vi "readBoardCounts.vi"(2 "input_portNum":i32=2, 3 "VISA resource name":refnum<visa-resource-name>="COM1") -> (0 "show_countInRange":bool=TRUE, 1 "show_messageOut":string="Port0 Usage Frequency: 017\nPort1 Usage Frequency: 017")   [LabVIEW 2011]
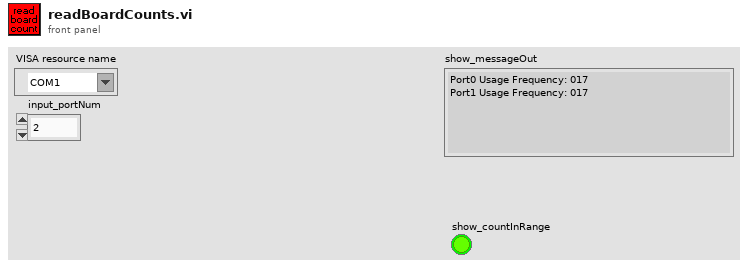
[diagram p1: front panel]
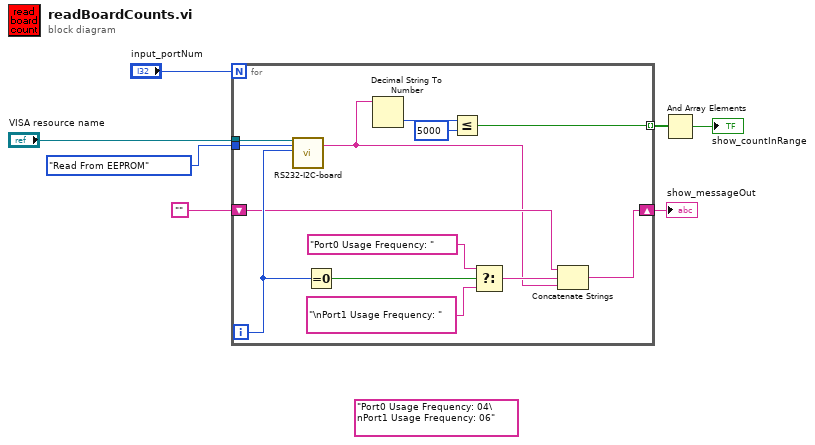
[diagram p0: block diagram]
diagram:
  (unwired) "Port0 Usage Frequency: 04\nPort1 Usage Frequency: 06"
  n1 = for {
    N: "input_portNum" -> [_]
    tunnel: "VISA resource name" -> [w20]
    tunnel: enum16{"Write to EEPROM", "Read From EEPROM"}."Read From EEPROM" ("Function") -> [w19]
    shift-right: [w12] -> w3
    shift-left: "" -> [w13]
    tunnel: [w8] -> w2 mode=indexing
    i -> [w18]
    n2 = call "RS232-I2C-board.vi"("VISA resource name"=w20, "Function"=w19, "Select channel"=w18) -> ("Read Data"=w11:string)  [unwired: 10 in, 6 out]
    n3 = Equal To 0?(x=w18) -> (x = 0?=w16:bool)
    n4 = Decimal String To Number(string=w11) -> (number=w10:i32)  [unwired: 2 in, 1 out]
    n5 = Less Or Equal?(x=w10, y=5000) -> (x <= y?=w8:bool)
    n6 = Select(t="Port0 Usage Frequency: ", s=w16, f="\nPort1 Usage Frequency: ") -> (s? t:f=w14:string)
    n7 = Concatenate Strings(w13, w14, w11) -> (w12:string)
  }
  "show_messageOut" <- w3
  n8 = And Array Elements(Boolean array=w2) -> (logical AND=→"show_countInRange":bool)
